vi "GET Row.vi"(8 "Error in":errorcluster caption="Error in (no error)", 10 "Row ID":u32=701, 11 "Table ID":u32=701) -> (0 "Error out":errorcluster, 3 "Rows Array JSON":string)   [LabVIEW 2018]
uses:
  Collect Param - Bool.vi
  <vilib>/httpClient/LabVIEWHTTPClient.lvlib
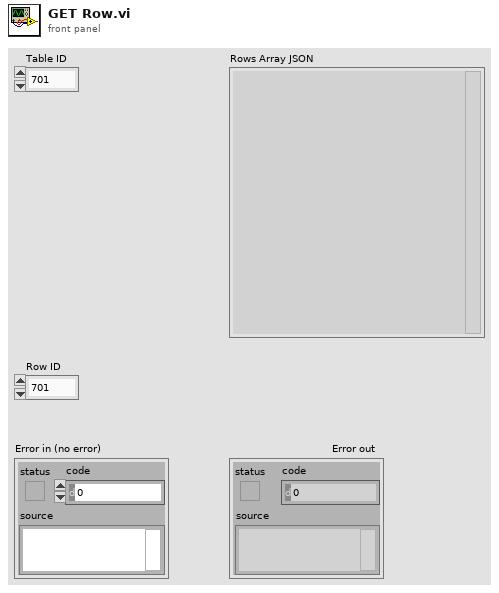
[diagram p1: front panel]
types:
  T1 = typedef "LabVIEWHTTPClient.lvlib/ClientHandle.ctl" = refnum<k1>
  T2 = typedef "Param.ctl" = cluster{"Param":string, "Value":string}
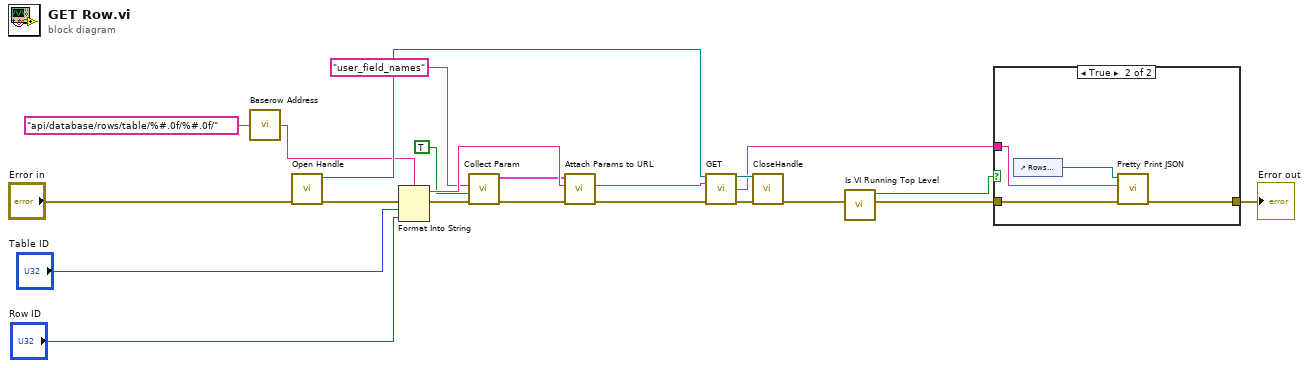
[diagram p0: block diagram]
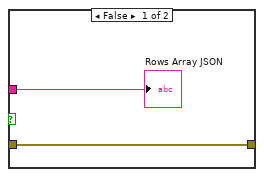
[diagram p2: hidden frame]
diagram:
  n1 = call "Baserow Address.vi"("Path"="api/database/rows/table/%#.0f/%#.0f/" ("url")) -> ("URL + Path"=w1:string)
  n2 = call "Open Handle.vi"("error in (no error)"="Error in") -> ("error out"=w19:errorcluster, "Refnum out"=w18:T1)  [unwired: 9 in]
  n3 = Format Into String(format string=w1, error in=w19, "Table ID", "Row ID") -> (resulting string=w22:string, error out=w14:errorcluster)  [unwired: 1 in]
  n4 = call-poly "Collect Param.vi"("Error in"=w14, "Value"=TRUE, "Param Name"="user_field_names") -> ("Error out"=w9:errorcluster, "Params Array Out"=w10:T2[])  [unwired: 7 in]
  n5 = call "Attach Params to URL.vi"("Error in"=w9, "URL"=w22, "Param array"=w10) -> ("Error out"=w11:errorcluster, "URL with params"=w12:string)  [unwired: 7 in]
  n6 = call <vilib>:"GET.vi"("client handle"=w18, "url"=w12, "error in (no error)"=w11) -> ("client handle out"=w20:T1, "body"=w7:string, "error out"=w8:errorcluster)  [unwired: 9 in, 1 out]
  n7 = call <vilib>:"CloseHandle.vi"("client handle"=w20, "error in (no error)"=w8) -> ("error out"=w6:errorcluster)  [unwired: 13 in]
  n8 = call "Is VI Running Top Level.vi"("Error in"=w6) -> ("Error out"=w5:errorcluster, "Top Level"=w4:bool)  [unwired: 9 in]
  n9 = case shown="True" w4 {
    tunnel: w7 -> [w23 w27]
    tunnel: w5 -> [w24 w26]
    tunnel: [w24 w25] -> w3
    frame False {
      "Rows Array JSON" <- w23
    }
    frame True {
      n10 = control-ref of="Rows Array JSON"() -> (w28:refnum<vi>)
      n11 = call "Pretty Print JSON.vi"("error in (no error)"=w26, "JSON in"=w27, "String in"=w28) -> ("error out"=w25:errorcluster)  [unwired: 8 in]
    }
  }
  "Error out" <- w3
